vi "Diag - SimpleMove.vi"() -> ()   [LabVIEW 2024]
uses:
  <vilib>/DAQmx/create/channels.llb/DAQmx Create Channel (DO-Digital Output).vi
panel:
  out "error out":errorcluster
  in  "physical channel":tag="NIUSBSALS/port0/line0:5"
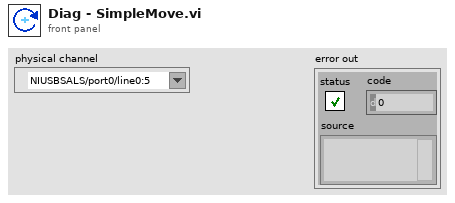
[diagram p1: front panel]
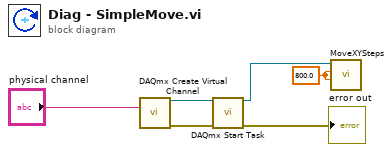
[diagram p0: block diagram]
diagram:
  w6 = 800.0 ("X Steps")
  n1 = call-poly <vilib>:"DAQmx Create Virtual Channel.vi"("lines"="physical channel") -> ("task out"=w4:refnum<k21>, "error out"=w1:errorcluster)  [unwired: 13 in]
  n2 = call <vilib>:"DAQmx Start Task.vi"("task/channels in"=w4, "error in"=w1) -> ("task out"=w3:refnum<k21>, "error out"=→"error out":errorcluster)  [unwired: 12 in]
  n3 = call "MoveXYSteps.vi"("Y Steps"=w6, "X Steps"=w6, "task in"=w3) -> ()  [unwired: 8 in, 1 out]
